vi "Trigger (DBL Array).vi"(2 "initialize":bool, 3 "trigger type":enum16{"rising", "falling", "either"}(ring), 5 "trigger signals":dbl[](array[numeric]) format="%.2f") -> (1 "triggered":bool[](array[boolean]))   [LabVIEW 2020, in "NI_AdvCtrl_nonlinear.lvlib"]
doc: "LabVIEW no longer supports this VI. You can obtain similar functionality by installing the LabVIEW Simulation Module.\n\nDetects changes of the input signal during the control or simulation process."
uses:
  <vilib>/addons/control/advanced/NI_AdvCtrl_nonlinear.lvlib
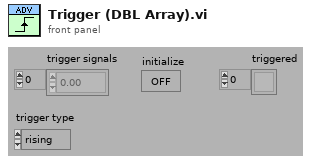
[diagram p1: front panel]
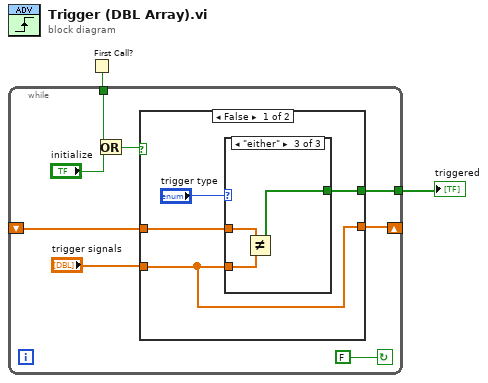
[diagram p0: block diagram]
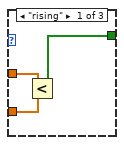
[diagram p2: hidden frame]
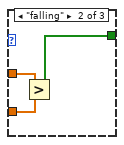
[diagram p3: hidden frame]
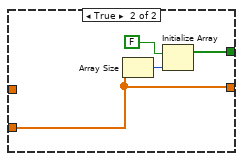
[diagram p4: hidden frame]
diagram:
  n1 = First Call?() -> (First Call?: T/F=w2:bool)
  n2 = while {
    tunnel: w2 -> [w6]
    tunnel: [w8] -> w1
    shift-left: _ -> [w9]
    shift-right: [w10] -> _
    stop <- FALSE continue-if-true
    n3 = Or(x=w6, y="initialize") -> (x .or. y?=w4:bool)
    n4 = case shown="False" w4 {
      tunnel: [w11 w27] -> w10
      tunnel: "trigger signals" -> [w11 w27]
      tunnel: w9 -> [w13 _]
      tunnel: [w12 w24] -> w8
      frame False {
        n5 = case shown="\"either\"" "trigger type" {
          tunnel: w13 -> [w17 w20 w23]
          tunnel: w11 -> [w16 w19 w22]
          tunnel: [w15 w18 w21] -> w12
          frame "rising" {
            n6 = Less?(x=w17, y=w16) -> (x < y?=w15:bool[])
          }
          frame "falling" {
            n7 = Greater?(x=w20, y=w19) -> (0:w18:bool[])
          }
          frame "either" {
            n8 = Not Equal?(x=w23, y=w22) -> (x != y?=w21:bool[])
          }
        }
      }
      frame True {
        n9 = Array Size(array=w27) -> (size(s)=w26:i32)
        n10 = Initialize Array(FALSE, w26) -> (w24:bool[])
      }
    }
  }
  "triggered" <- w1
